vi "Control Loop.vi"(8 "error in (no error)":errorcluster, 10 "notifier out":refnum<notifier>, 11 "Message Queues":T1) -> (0 "error out":errorcluster)   [LabVIEW 2026, in "Control.lvlib"]
uses:
  Control.lvlib
  support/Message Queue/All Message Queues.ctl
  support/Message Queue/Message Cluster.ctl
  controls/NotifierAndDataQueue.ctl
  controls/WaveformChartData.ctl
  Acquisition/Hardware Configuration.ctl
  Acquisition/Acquisition State.ctl
  <vilib>/DAQmx/write.llb/DAQmx Write (Analog 1D DBL NChan 1Samp).vi
  <vilib>/DAQmx/write.llb/DAQmx Write (Digital 1D Bool 1Chan 1Samp).vi
  support/Message Queue/Enqueue Message (Single).vi
  <vilib>/DAQmx/miscellaneous.llb/DAQmx Fill In Error Info.vi
  <vilib>/Utility/error.llb/Error Cluster From Error Code.vi
  <vilib>/ErrorRing/Error Ring.xnode
  Acquisition/Acquisition.lvlib
  support/Message Queue/Message Queue.lvlib
  Settings/Settings.lvlib
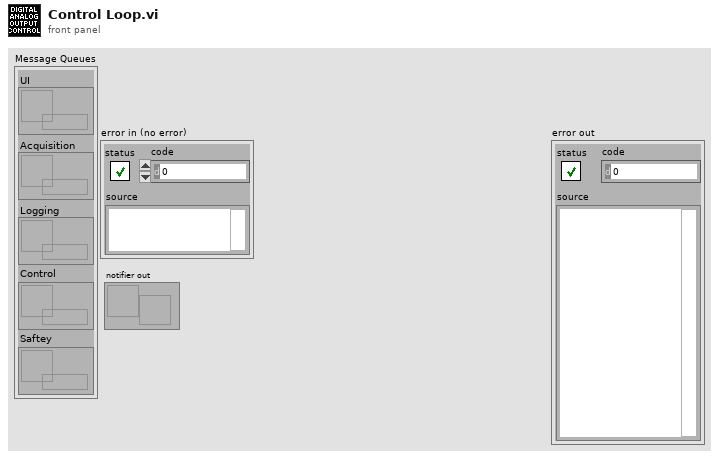
[diagram p1: front panel]
types:
  T1 = typedef "Message Queue.lvlib/All Message Queues.ctl" = cluster{"UI":refnum<queue>, "Acquisition":refnum<queue>, "Logging":refnum<queue>, "Control":refnum<queue>, "Saftey":refnum<queue>}
  T2 = typedef "Acquisition.lvlib/Hardware Configuration.ctl" = cluster{"Analog Out array":dbl[], "Initialize Flag":bool, "Saftey Table Display":refnum<vi>, "Torque&Force":waveform(dbl)[][], "Calibration Data":waveform(dbl)[], "2D":dbl[][], "Analog In Task":refnum<k21>, "Digital In Task":refnum<k21>, "Analog Out Task":refnum<k21>, "Digital Out Task":refnum<k21>, "Digital Out Array":bool[], "Current Cycle Count":refnum<vi>, "Cycle Count":u64, "Headers":string[], "Sweep Interval":u64, "Delay":u64, "TestConfigDisplay":refnum<vi>, "50psi Conversion":dbl[], "1245N15 Conversion":dbl[], "MX06F Conversion":dbl[], "# of Test Cycles":u64, "60psi Conversion":dbl[], "100psi Conversion":dbl[], "200psi Conversion":dbl[], "1000psi Conversion":dbl[], "2000psi Conversion":dbl[], "5000psi Conversion":dbl[], "MX09F Conversion":dbl[], "MX19F Conversion":dbl[], "DUT VALVE POSITION":refnum<vi>, "INTAKE VALVE POSITION":refnum<vi>, "Table Control":refnum<vi>, "Table Control":string[][], "Max Vacuum":dbl, "RPM Ramp Ref":refnum<vi>, "Free Air Flow Ref":refnum<vi>, "Press Stable Ref":refnum<vi>, "Press Decay Ref":refnum<vi>}
  T3 = typedef "Acquisition.lvlib/Acquisition State.ctl" = enum16{"Idle", "Acquiring"}
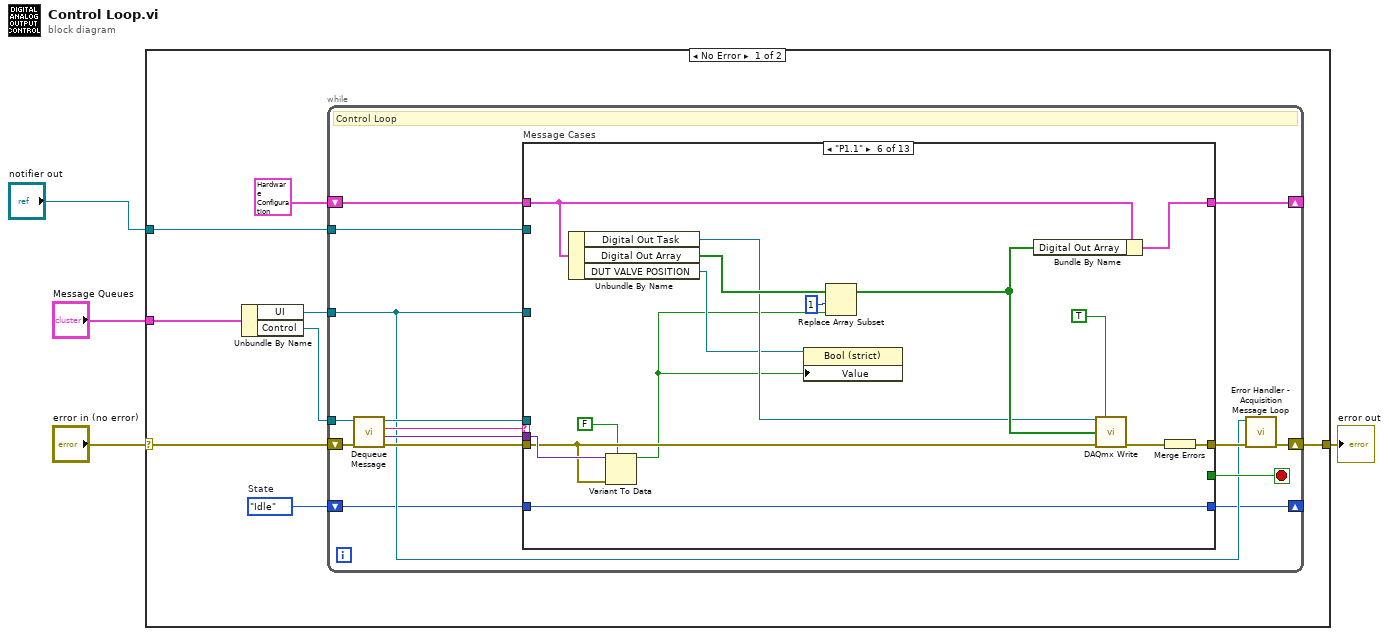
[diagram p0: block diagram]
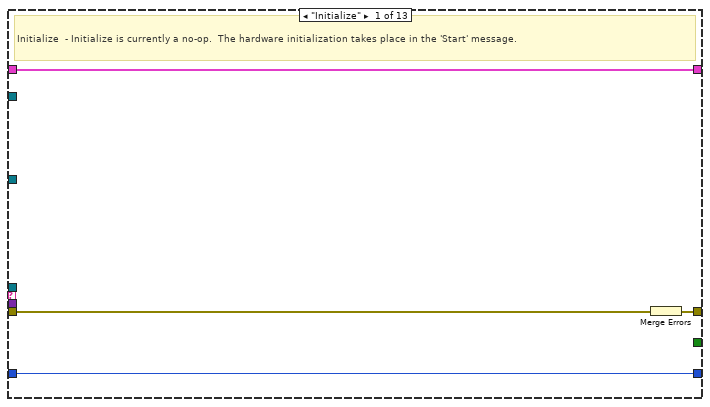
[diagram p2: hidden frame]
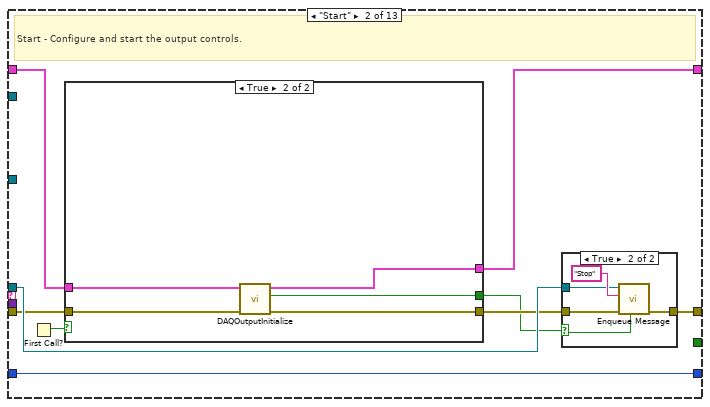
[diagram p3: hidden frame]
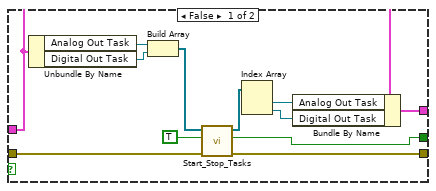
[diagram p4: hidden frame]
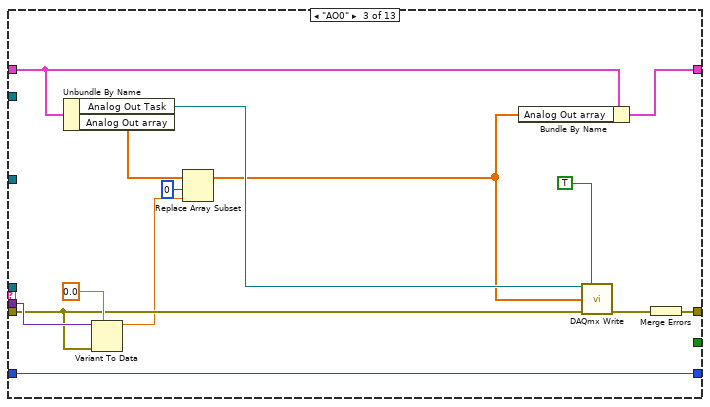
[diagram p6: hidden frame]
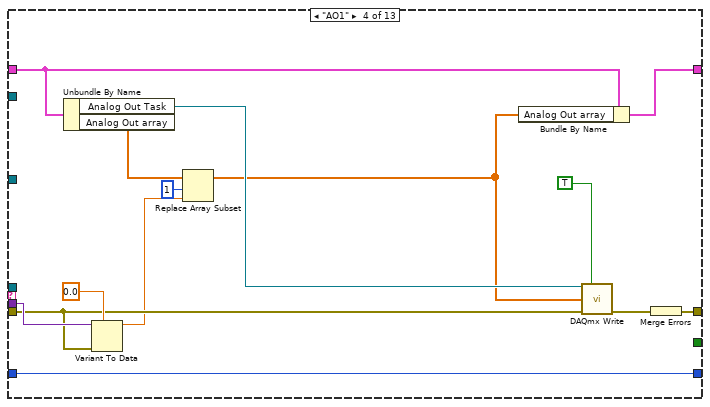
[diagram p7: hidden frame]
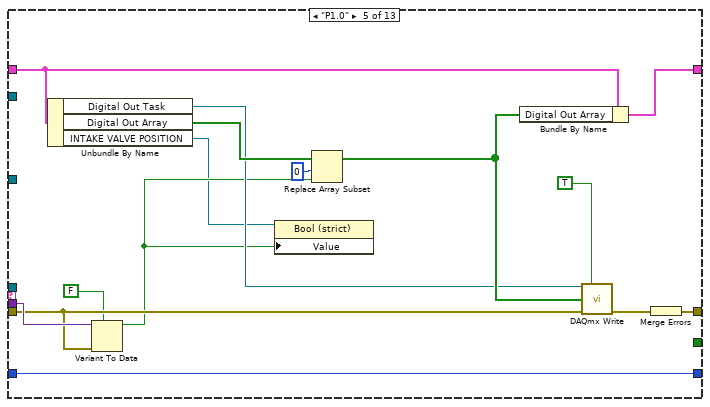
[diagram p8: hidden frame]
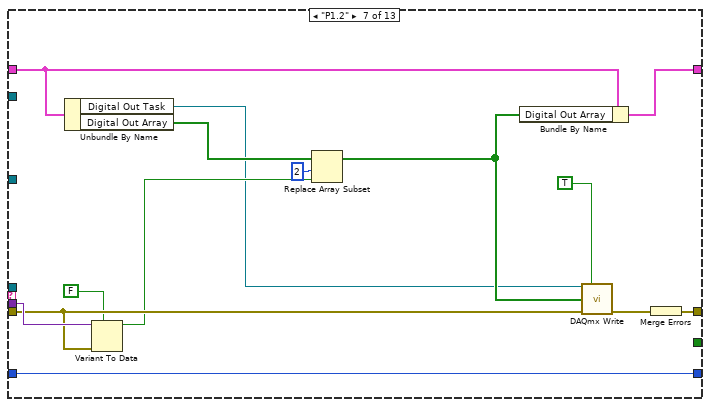
[diagram p9: hidden frame]
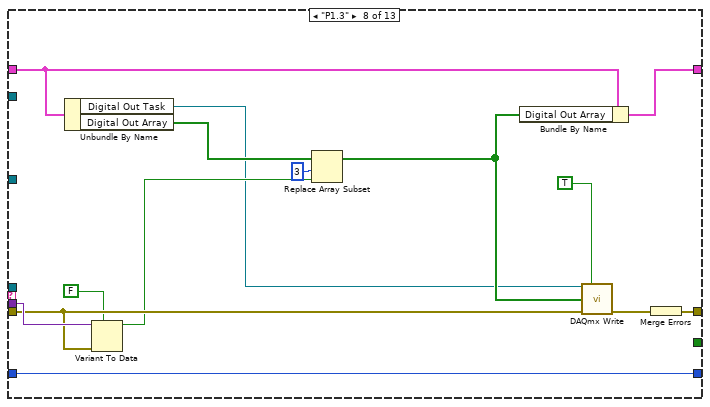
[diagram p10: hidden frame]
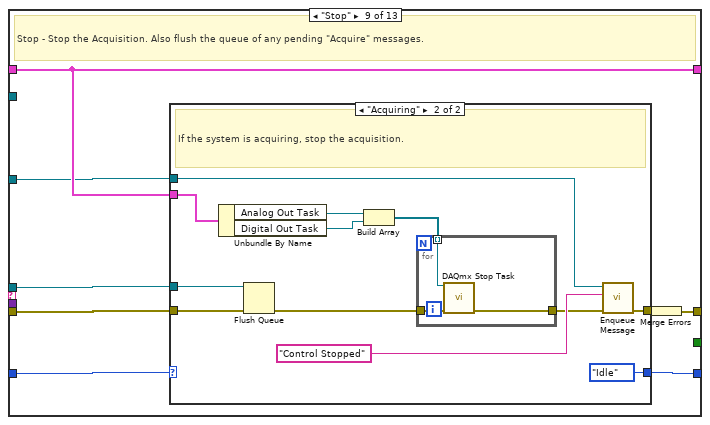
[diagram p11: hidden frame]
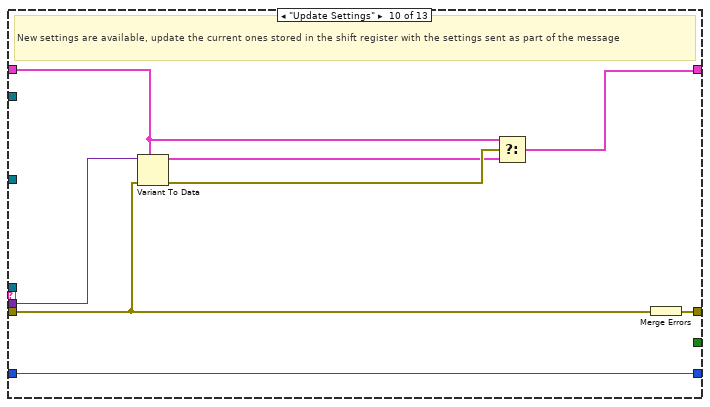
[diagram p13: hidden frame]
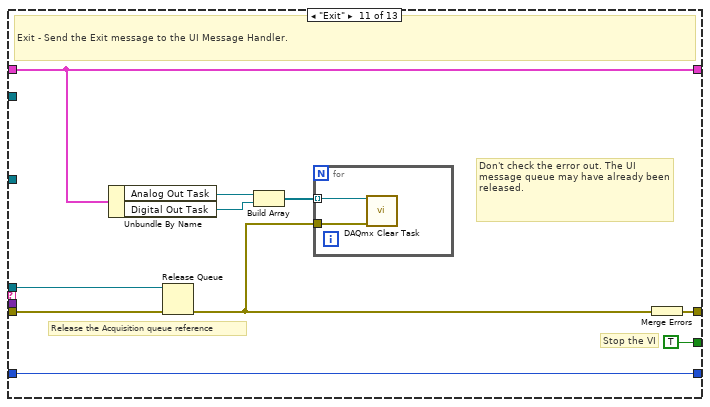
[diagram p14: hidden frame]
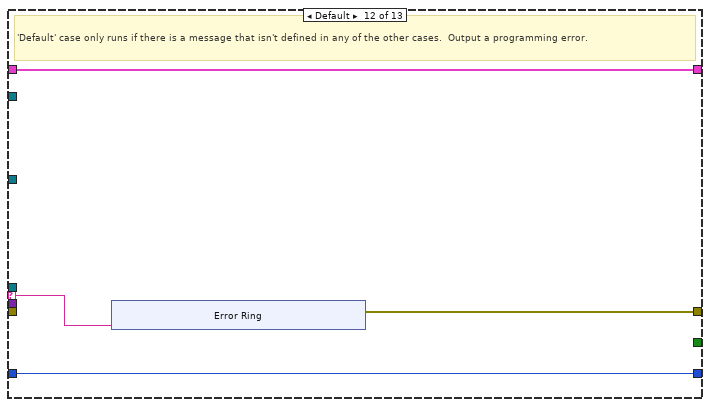
[diagram p15: hidden frame]
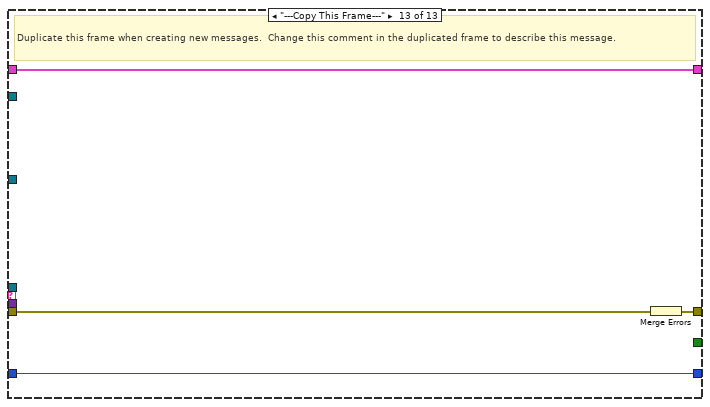
[diagram p16: hidden frame]
diagram:
  n1 = case shown="No Error" "error in (no error)" {
    selector: "error in (no error)" -> [w8 w210]
    tunnel: "Message Queues" -> [w12 _]
    tunnel: [w10 w210] -> w3
    tunnel: "notifier out" -> [w6 _]
    frame No Error {
      w5 = Acquisition_State."Idle"  # State
      n2 = Unbundle By Name(w12) -> ("UI"=w7:refnum<queue>, "Control"=w11:refnum<queue>)
      n3 = while {
        tunnel: w11 -> [w19]
        shift-right: [w26] -> _
        shift-left: T2 {"Analog Out array"=[], "Initialize Flag"=FALSE, "Saftey Table Display"=refnum, "Torque&Force"=[], "Calibration Data"=[], "2D"=[], "Analog In Task"="", "Digital In Task"="", "Analog Out Task"="", "Digital Out Task"="", "Digital Out Array"=[], "Current Cycle Count"=refnum, "Cycle Count"=0, "Headers"=[], "Sweep Interval"=0, "Delay"=0, "TestConfigDisplay"=refnum, "50psi Conversion"=[], "1245N15 Conversion"=[], "MX06F Conversion"=[], "# of Test Cycles"=0, "60psi Conversion"=[], "100psi Conversion"=[], "200psi Conversion"=[], "1000psi Conversion"=[], "2000psi Conversion"=[], "5000psi Conversion"=[], "MX09F Conversion"=[], "MX19F Conversion"=[], "DUT VALVE POSITION"=refnum, "INTAKE VALVE POSITION"=refnum, "Table Control"=refnum, "Table Control"=[], "Max Vacuum"=0.0, "RPM Ramp Ref"=refnum, "Free Air Flow Ref"=refnum, "Press Stable Ref"=refnum, "Press Decay Ref"=refnum} ("Data Cluster") -> [w27]
        shift-right: [w16] -> w10
        shift-left: w8 -> [w24]
        tunnel: w7 -> [w15]
        tunnel: w6 -> [w18]
        shift-right: [w13] -> _
        shift-left: w5 -> [w14]
        stop <- w25 stop-if-true
        # "Control Loop"
        n4 = call "Dequeue Message.vi"("error in (no error)"=w24, "Message Queue"=w19) -> ("error out"=w23:errorcluster, "Message Data"=w21:variant, "Message"=w22:string, "dup Message Queue"=w20:refnum<queue>)  [unwired: 6 in]
        n5 = case "Message Cases" shown="\"P1.1\"" w22 {
          selector: w22 -> [_ _ _ _ _ _ _ _ _ _ _ w197 _]
          tunnel: w20 -> [_ w36 _ _ _ _ _ _ w154 _ w189 _ _]
          tunnel: w23 -> [w30 w33 w71 w85 w102 w117 w131 w145 w156 w176 w190 _ w209]
          tunnel: [w31 w37 w77 w91 w106 w121 w135 w149 w157 w182 w191 w196 w207] -> w17
          tunnel: w27 -> [w28 w39 w66 w80 w98 w113 w126 w140 w155 w178 w184 w198 w208]
          tunnel: [w28 w38 w65 w79 w97 w112 w125 w139 w155 w177 w184 w198 w208] -> w26
          tunnel: [_ _ _ _ _ _ _ _ _ _ TRUE _ _] -> w25
          tunnel: w21 -> [_ _ w75 w89 w104 w119 w133 w147 _ w181 _ _ _]
          tunnel: w15 -> [_ _ _ _ _ _ _ _ w153 _ _ _ _]
          tunnel: w18 -> [_ _ _ _ _ _ _ _ _ _ _ _ _]
          tunnel: w14 -> [w29 w40 w76 w90 w105 w120 w134 w148 w152 w175 w188 w195 w206]
          tunnel: [w29 w40 w76 w90 w105 w120 w134 w148 w151 w175 w188 w195 w206] -> w13
          frame "Initialize" {
            # "Initialize  - Initialize is currently a no-op.  The hardware initialization takes place in the 'Start' message."
            n6 = Merge Errors(w30) -> (w31:errorcluster)
          }
          frame "Start" {
            # "Start - Configure and start the output controls."
            n7 = First Call?() -> (First Call?: T/F=w32:bool)
            n8 = case shown="True" w32 {
              tunnel: w39 -> [w45 w53]
              tunnel: [w44 w57] -> w38
              tunnel: [w50 w56] -> w35
              tunnel: [w43 w55] -> w34
              tunnel: w33 -> [w51 w54]
              frame False {
                n9 = Unbundle By Name(w45) -> ("Analog Out Task"=w49:refnum<k21>, "Digital Out Task"=w48:refnum<k21>)
                n10 = Build Array(w49, w48) -> (w47:refnum<k21>[])
                n11 = call "Start_Stop_Tasks.vi"("error in"=w51, "Start/Stop Task"=TRUE, "Tasks In"=w47) -> ("error out"=w50:errorcluster, "error?"=w43:bool, "Tasks Out"=w46:refnum<k21>[])  [unwired: 6 in]
                n12 = Index Array(array=w46) -> (element #1=w42:refnum<k21>, element #2=w41:refnum<k21>)  [unwired: 2 in]
                n13 = Bundle By Name(cluster=w45, "Analog Out Task"=w42, "Digital Out Task"=w41) -> (w44:T2)
              }
              frame True {
                n14 = call "DAQOutputInitialize.vi"("error in (no error)"=w54, "Data Cluster in"=w53) -> ("error out"=w56:errorcluster, "error?"=w55:bool, "Data Cluster out"=w57:T2)  [unwired: 7 in]
              }
            }
            n15 = case shown="True" w34 {
              selector: w34 -> [_ w59]
              tunnel: w35 -> [w58 w60]
              tunnel: [w58 w62] -> w37
              tunnel: w36 -> [_ w61]
              frame False {
              }
              frame True {
                n16 = call-poly "Enqueue Message.vi"("Priority Message? (F)"=w59, "error in (no error)"=w60, "Message"="Stop", "Message Queue"=w61) -> ("error out"=w62:errorcluster)  [unwired: 6 in, 1 out]
              }
            }
          }
          frame "AO0" {
            n17 = Unbundle By Name(w66) -> ("Analog Out Task"=w73:refnum<k21>, "Analog Out array"=w68:dbl[])
            n18 = Variant To Data(error in=w71, type=0.0, Variant=w75) -> (data=w69:dbl)  [unwired: 1 out]
            n19 = Replace Array Subset(array=w68, new element=w69, index=0) -> (w64:dbl[])
            n20 = Bundle By Name(cluster=w66, "Analog Out array"=w64) -> (w65:T2)
            n21 = call-poly <vilib>:"DAQmx Write.vi"("task/channels in"=w73, "auto start"=TRUE, "data"=w64, "error in"=w71) -> ("error out"=w70:errorcluster)  [unwired: 9 in, 2 out]
            n22 = Merge Errors(w70) -> (w77:errorcluster)
          }
          frame "AO1" {
            n23 = Unbundle By Name(w80) -> ("Analog Out Task"=w87:refnum<k21>, "Analog Out array"=w82:dbl[])
            n24 = Variant To Data(error in=w85, type=0.0, Variant=w89) -> (data=w83:dbl)  [unwired: 1 out]
            n25 = Replace Array Subset(array=w82, new element=w83, index=1) -> (w78:dbl[])
            n26 = Bundle By Name(cluster=w80, "Analog Out array"=w78) -> (w79:T2)
            n27 = call-poly <vilib>:"DAQmx Write.vi"("task/channels in"=w87, "auto start"=TRUE, "data"=w78, "error in"=w85) -> ("error out"=w84:errorcluster)  [unwired: 9 in, 2 out]
            n28 = Merge Errors(w84) -> (w91:errorcluster)
          }
          frame "P1.0" {
            n29 = Unbundle By Name(w98) -> ("Digital Out Task"=w94:refnum<k21>, "Digital Out Array"=w100:bool[], "INTAKE VALVE POSITION"=w92:refnum<vi>)
            n30 = Variant To Data(error in=w102, type=FALSE, Variant=w104) -> (data=w93:bool)  [unwired: 1 out]
            n31 = property class="Bool (strict)"(reference=w92, "Value"=w93) -> ()  [unwired: 1 in, 2 out]
            n32 = Replace Array Subset(array=w100, new element=w93, index=0) -> (w96:bool[])
            n33 = Bundle By Name(cluster=w98, "Digital Out Array"=w96) -> (w97:T2)
            n34 = call-poly <vilib>:"DAQmx Write.vi"("task/channels in"=w94, "auto start"=TRUE, "data"=w96, "error in"=w102) -> ("error out"=w101:errorcluster)  [unwired: 9 in, 2 out]
            n35 = Merge Errors(w101) -> (w106:errorcluster)
          }
          frame "P1.1" {
            n36 = Unbundle By Name(w113) -> ("Digital Out Task"=w109:refnum<k21>, "Digital Out Array"=w115:bool[], "DUT VALVE POSITION"=w108:refnum<vi>)
            n37 = Variant To Data(error in=w117, type=FALSE, Variant=w119) -> (data=w107:bool)  [unwired: 1 out]
            n38 = property class="Bool (strict)"(reference=w108, "Value"=w107) -> ()  [unwired: 1 in, 2 out]
            n39 = Replace Array Subset(array=w115, new element=w107, index=1) -> (w111:bool[])
            n40 = Bundle By Name(cluster=w113, "Digital Out Array"=w111) -> (w112:T2)
            n41 = call-poly <vilib>:"DAQmx Write.vi"("task/channels in"=w109, "auto start"=TRUE, "data"=w111, "error in"=w117) -> ("error out"=w116:errorcluster)  [unwired: 9 in, 2 out]
            n42 = Merge Errors(w116) -> (w121:errorcluster)
          }
          frame "P1.2" {
            n43 = Unbundle By Name(w126) -> ("Digital Out Task"=w122:refnum<k21>, "Digital Out Array"=w128:bool[])
            n44 = Variant To Data(error in=w131, type=FALSE, Variant=w133) -> (data=w129:bool)  [unwired: 1 out]
            n45 = Replace Array Subset(array=w128, new element=w129, index=2) -> (w124:bool[])
            n46 = Bundle By Name(cluster=w126, "Digital Out Array"=w124) -> (w125:T2)
            n47 = call-poly <vilib>:"DAQmx Write.vi"("task/channels in"=w122, "auto start"=TRUE, "data"=w124, "error in"=w131) -> ("error out"=w130:errorcluster)  [unwired: 9 in, 2 out]
            n48 = Merge Errors(w130) -> (w135:errorcluster)
          }
          frame "P1.3" {
            n49 = Unbundle By Name(w140) -> ("Digital Out Task"=w136:refnum<k21>, "Digital Out Array"=w142:bool[])
            n50 = Variant To Data(error in=w145, type=FALSE, Variant=w147) -> (data=w143:bool)  [unwired: 1 out]
            n51 = Replace Array Subset(array=w142, new element=w143, index=3) -> (w138:bool[])
            n52 = Bundle By Name(cluster=w140, "Digital Out Array"=w138) -> (w139:T2)
            n53 = call-poly <vilib>:"DAQmx Write.vi"("task/channels in"=w136, "auto start"=TRUE, "data"=w138, "error in"=w145) -> ("error out"=w144:errorcluster)  [unwired: 9 in, 2 out]
            n54 = Merge Errors(w144) -> (w149:errorcluster)
          }
          frame "Stop" {
            # "Stop - Stop the Acquisition. Also flush the queue of any pending \"Acquire\" messages."
            n55 = case shown="\"Acquiring\"" w152 {
              selector: w152 -> [w159 _]
              tunnel: w156 -> [w158 w171]
              tunnel: w155 -> [_ w163]
              tunnel: w154 -> [_ w170]
              tunnel: w153 -> [_ w169]
              tunnel: [w159 Acquisition_State."Idle" ("State")] -> w151
              tunnel: [w158 w168] -> w150
              frame "Idle", Default {
                # "The system is already idle. Ignore the \"Stop\" message."
              }
              frame "Acquiring" {
                # "If the system is acquiring, stop the acquisition."
                n56 = Unbundle By Name(w163) -> ("Analog Out Task"=w162:refnum<k21>, "Digital Out Task"=w161:refnum<k21>)
                n57 = Flush Queue(queue=w170, error in (no error)=w171) -> (error out=w165:errorcluster)  [unwired: 2 out]
                n58 = Build Array(w162, w161) -> (w160:refnum<k21>[])
                n59 = for {
                  tunnel: w165 -> [w174]
                  tunnel: [w172] -> w164
                  tunnel: w160 -> [w173] mode=indexing
                  n60 = call <vilib>:"DAQmx Stop Task.vi"("task/channels in"=w173, "error in"=w174) -> ("error out"=w172:errorcluster)  [unwired: 12 in, 1 out]
                }
                n61 = call-poly "Enqueue Message.vi"("error in (no error)"=w164, "Message"="Control Stopped", "Message Queue"=w169) -> ("error out"=w168:errorcluster)  [unwired: 7 in, 1 out]
              }
            }
            n62 = Merge Errors(w150) -> (w157:errorcluster)
          }
          frame "Update Settings" {
            # "New settings are available, update the current ones stored in the shift register with the settings sent as part of the message"
            n63 = Variant To Data(error in=w176, type=w178, Variant=w181) -> (data=w179:T2, error out=w180:errorcluster)
            n64 = Select(t=w178, s=w180, f=w179) -> (s? t:f=w177:T2)
            n65 = Merge Errors(w176) -> (w182:errorcluster)
          }
          frame "Exit" {
            # "Don't check the error out. The UI message queue may have already been released."
            # "Release the Acquisition queue reference"
            # "Stop the VI"
            # "Exit - Send the Exit message to the UI Message Handler."
            n66 = Unbundle By Name(w184) -> ("Analog Out Task"=w187:refnum<k21>, "Digital Out Task"=w186:refnum<k21>)
            n67 = Release Queue(queue=w189, error in (no error)=w190) -> (error out=w183:errorcluster)  [unwired: 1 in, 2 out]
            n68 = Build Array(w187, w186) -> (w185:refnum<k21>[])
            n69 = for {
              tunnel: w183 -> [w193]
              tunnel: w185 -> [w194] mode=indexing
              n70 = call <vilib>:"DAQmx Clear Task.vi"("task in"=w194, "error in"=w193) -> ()  [unwired: 13 in, 1 out]
            }
            n71 = Merge Errors(w183) -> (w191:errorcluster)
          }
          frame Default {
            # "'Default' case only runs if there is a message that isn't defined in any of the other cases.  Output a programming error."
            n72 = xnode "Error Ring"("parameter 0"=w197) -> ("error out"=w196:errorcluster)
          }
          frame "---Copy This Frame---" {
            # "Duplicate this frame when creating new messages.  Change this comment in the duplicated frame to describe this message."
            n73 = Merge Errors(w209) -> (w207:errorcluster)
          }
        }
        n74 = call "Error Handler - Acquisition Message Loop.vi"("error in (no error)"=w17, "Message Queue"=w15) -> ("dup error in"=w16:errorcluster)  [unwired: 8 in, 1 out]
      }
    }
    frame Error {
    }
  }
  "error out" <- w3
